vi "Get Tags - Force Data Conversion.vi"(7 "Force Data Conversion? (F)":bool, 8 "error in (no error)":errorcluster, 9 "default value":variant, 10 "key":string, 11 "Map":map{string, variant}(c390)) -> (0 "error out":errorcluster, 1 "value":variant, 4 "found?":bool)   [LabVIEW 2023, in "uLib.lvlib" / "uData.lvclass"]
doc: "This method operates on pre-queried tags and it has an option to force explicit data conversion if data types are not the same.\nIf not enabled, it defaults to the same behavior as the \"Get Tag.vi\" method.\n\n<B>This is still experimental.</B> Use with caution."
uses:
  uData.lvclass
  <vilib>/Utility/Data Type/Type Definitions/Data Type.ctl
  uData.lvclass/uData.ctl
  <vilib>/Utility/Data Type/NI_Data Type.lvlib
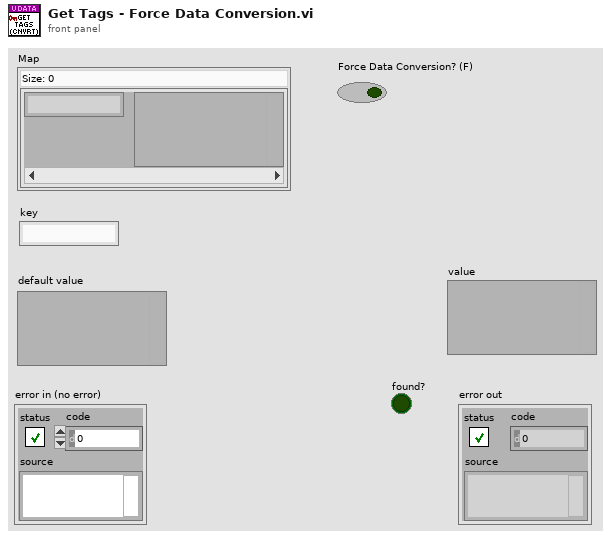
[diagram p1: front panel]
types:
  T1 = typedef "NI_Data Type.lvlib/Data Type.ctl" = enum8{"Invalid Type", "Void", "I8", "I16", "I32", "I64", "U8", "U16", "U32", "U64", "Single Float", "Double Float", "Extended Float", "Single Complex", "Double Complex", "Extended Complex", "Enum U8", "Enum U16", "Enum U32", "Enum U64", "Single Float With Unit", "Double Float With Unit", "Extended Float With Unit", "Single Complex with Unit", "Double Complex with Unit", "Extended Complex with Unit", "Boolean", "String", "Path", "Picture", "Tag", "Array", "Cluster", "Variant", "LV Variant", "Waveform", "Timestamp", "Digital Waveform", "Digital Data", "ExpressData", "Refnum", "External Data", "VI", "Poly VI", "LabVIEW Class Instance", "Fixed Point", "Set Collection", "Map Collection"}
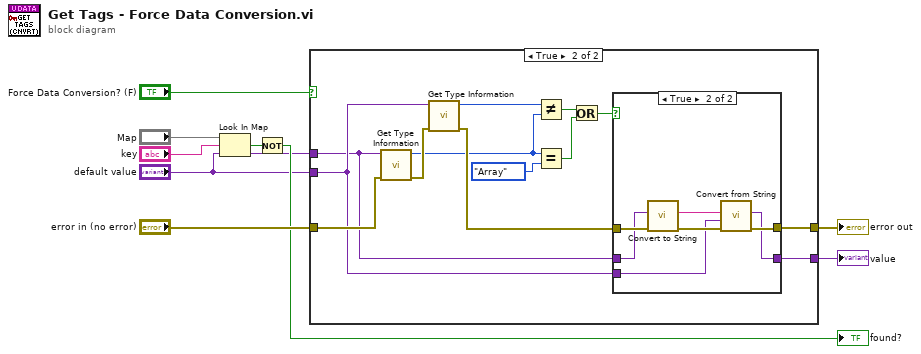
[diagram p0: block diagram]
diagram:
  n1 = Look In Map(map="Map", key="key", default value="default value") -> (key not found?=w2:bool, value=w3:variant)
  n2 = Not(x=w2) -> (.not. x?=→"found?":bool)
  n3 = case shown="True" "Force Data Conversion? (F)" {
    tunnel: "error in (no error)" -> [w12 w25]
    tunnel: [w12 w24] -> w7
    tunnel: [w11 w23] -> w6
    tunnel: "default value" -> [_ w22]
    tunnel: w3 -> [w11 w21]
    frame False {
    }
    frame True {
      n4 = call <vilib>:"Get Type Information.vi"("error in (no error)"=w25, "variant"=w21) -> ("error out"=w20:errorcluster, "type"=w15:T1)  [unwired: 5 in, 3 out]
      n5 = call <vilib>:"Get Type Information.vi"("error in (no error)"=w20, "variant"=w22) -> ("error out"=w18:errorcluster, "type"=w19:T1)  [unwired: 5 in, 3 out]
      n6 = Not Equal?(x=w19, y=w15) -> (x != y?=w17:bool)
      n7 = Equal?(x=w15, y=Data_Type."Array") -> (x = y?=w14:bool)
      n8 = Or(x=w17, y=w14) -> (x .or. y?=w16:bool)
      n9 = case shown="True" w16 {
        tunnel: w18 -> [w27 w33]
        tunnel: [w27 w34] -> w24
        tunnel: w21 -> [w26 w32]
        tunnel: [w26 w29] -> w23
        tunnel: w22 -> [_ w28]
        frame False {
        }
        frame True {
          n10 = call "Convert to String.vi"("error in (no error)"=w33, "data"=w32) -> ("error out"=w31:errorcluster, "String"=w30:string)  [unwired: 8 in]
          n11 = call "Convert from String.vi"("error in (no error)"=w31, "data type"=w28, "String"=w30) -> ("error out"=w34:errorcluster, "data"=w29:variant)  [unwired: 7 in]
        }
      }
    }
  }
  "error out" <- w7
  "value" <- w6
